vi "RT Main Test.vi"() -> ()   [LabVIEW 2020]
uses:
  <vilib>/Platform/TimedLoop/XDataNode/timing_clust.ctl
  <vilib>/Platform/TimedLoop/XDataNode/nitl_modes.ctl
  <vilib>/Platform/TimedLoop/XDataNode/wakeup.ctl
  Type Definitions/Payload Class.ctl
  Type Definitions/Enumerated Constants/Software Monitor.ctl
  Type Definitions/Queue Monitor.ctl
  Type Definitions/Telemetry TCP State.ctl
  Type Definitions/Enum - System State.ctl
  Type Definitions/Data Frame.ctl
  Type Definitions/Data Frame Header.ctl
  SubVIs/Compute CRC32.vi
  <vilib>/platform/TimedLoop/XDataNode/XDataNode.xnode
  <vilib>/Platform/TimedLoop/XDataNode/XDNodeRunTimeDep.lvlib
panel:
  out "error out":errorcluster
  out "Remote Address":string
  out "Remote Port":u16
  out "Frames Sent":i32
  out "Bytes Sent":i32
  out "Is Connected":bool
  out "Linux Standard Out":string
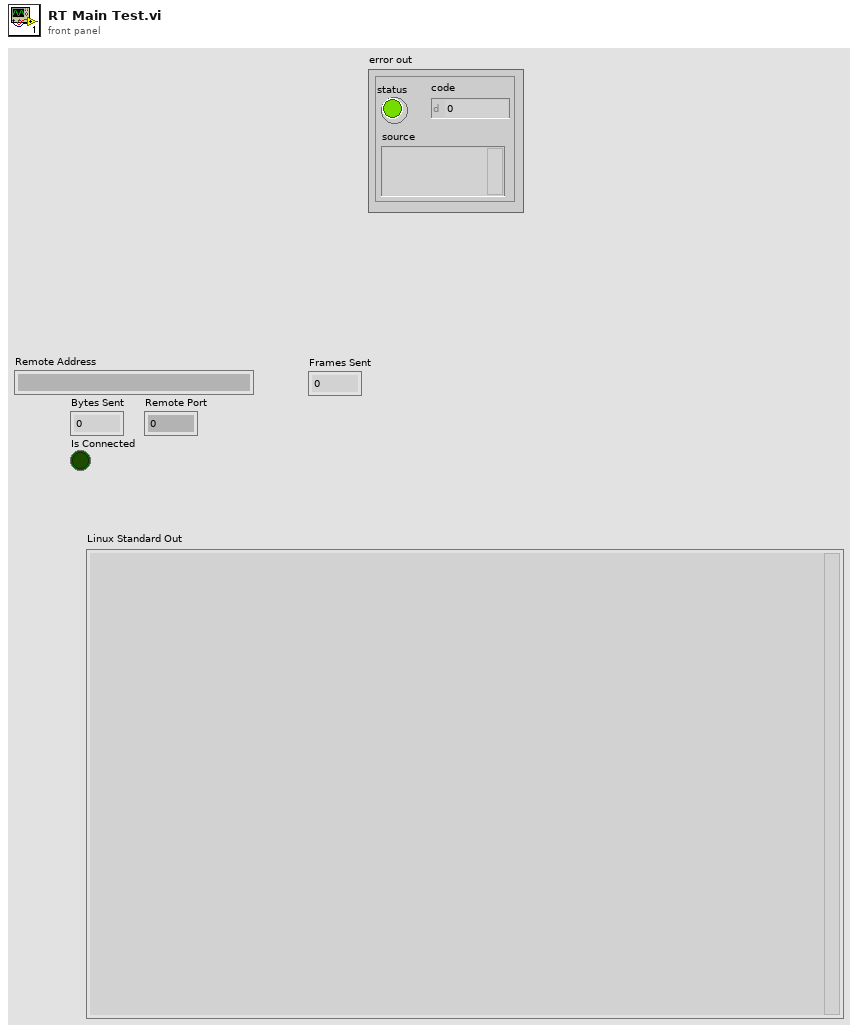
[diagram p1: front panel]
types:
  T1 = typedef "XDNodeRunTimeDep.lvlib/timing_clust.ctl" = cluster{"Expected End [f-1]":u64, "Actual End [f-1]":u64, "Finished Late? [f-1]":bool, "Expected End [i-1]":u64, "Actual End [i-1]":u64, "Finished Late? [i-1]":bool, "Expected Start [i]":u64, "Actual Start [i]":u64, "Expected Start [f]":u64, "Actual Start [f]":u64, "Source Name":string, "Structure Name":string, "Period":i64, "Deadline":i64, "Offset":i64, "Start":i64, "Priority":i32, "Timeout":i32, "Mode":T2, "Wakeup Reason":T3, "Error":errorcluster, "Source Type":string, "Secondary Source Type":string, "Global End Time":u64, "Global Start Time":u64, "Frame Duration":u64, "Iteration Duration":u64, "Assigned CPU":i32, "I/O Scan Engine Mode":u32}
  T2 = typedef "XDNodeRunTimeDep.lvlib/nitl_modes.ctl" = enum32{"No Change", "Process missed periods, maintain original phase", "Discard missed periods, maintain original phase", "Process missed periods, ignore original phase", "Discard missed periods, ignore original phase"}
  T3 = typedef "XDNodeRunTimeDep.lvlib/wakeup.ctl" = enum32{"Normal", "Aborted", "Asynchronous wakeup", "Timing source error", "Timed loop error", "Timeout"}
  T4 = typedef "Software Monitor.ctl" = enum16{"Internet Connection Monitor", "CPU Monitor", "Archive Monitor", "Memory Monitor", "Queue Monitor", "RTOS Update", "RTOS Monitor"}
  T5 = typedef "Payload Class.ctl" = enum16{"System State", "Parameters", "Metadata", "Software Monitor", "Data", "Commands"}
  T6 = typedef "Queue Monitor.ctl" = cluster{"Queue Name":string, "Max Queue Size":i32, "Pending Remove":i32, "Pending Insert":i32, "Elements in Queue":i32}
  T7 = typedef "Data Frame.ctl" = cluster{"Frame Header":T8, "Payload":string, "CRC":u32}
  T8 = typedef "Data Frame Header.ctl" = cluster{"Sync":u32, "Time":dbl, "Nanosecond Counter":i64, "Payload Class":T5, "Payload ID":u16, "Counter":u32, "Options":u32, "Source":i32, "Destination":i32}
  T9 = typedef "Enum - System State.ctl" = enum16{"System Time", "Telemetry TCP State", "Writeable Drive State", "Command TCP State", "Network Adapter State", "Discovery Engine State", "Disk State"}
  T10 = typedef "Telemetry TCP State.ctl" = cluster{"Is Connected":bool, "Remote Address":string, "Remote Port":u16, "Total Frames Sent":i32, "Total Bytes Sent":i32}
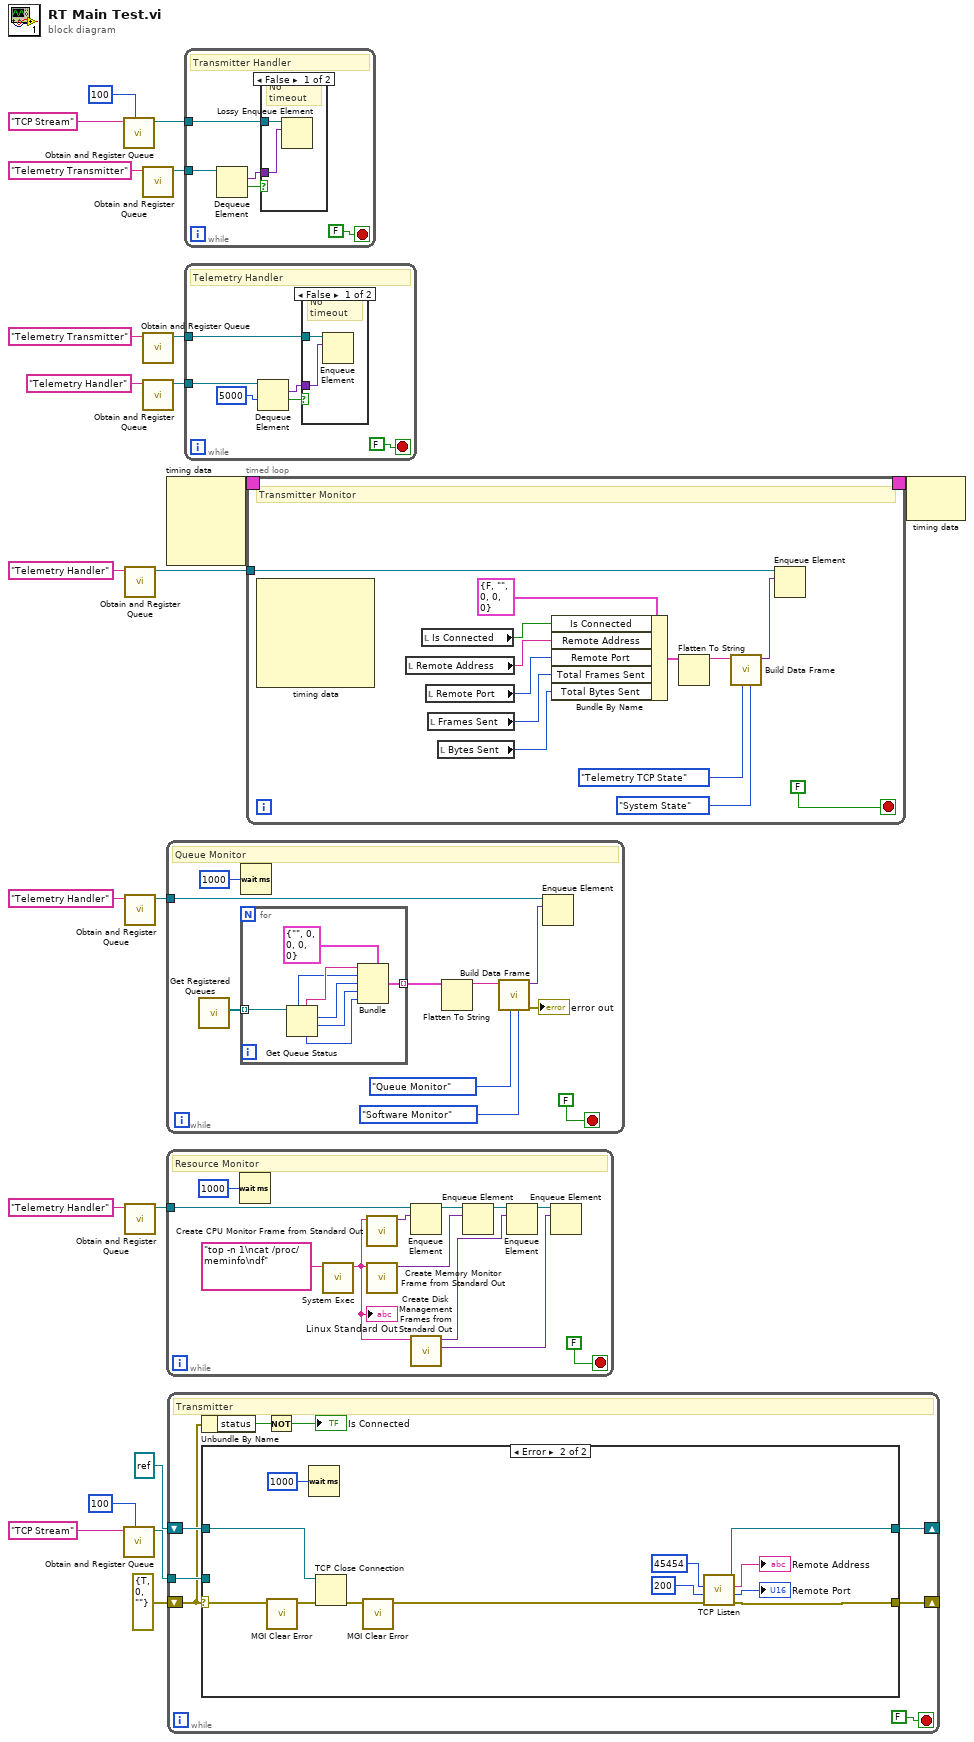
[diagram p0: block diagram]
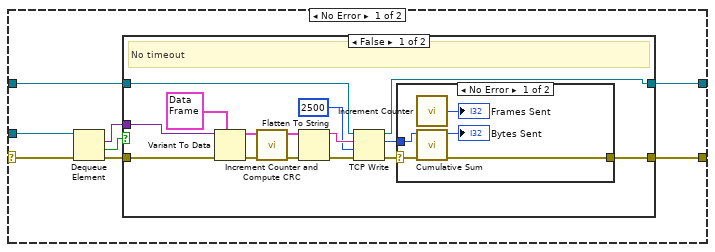
[diagram p3: hidden frame]
diagram:
  n1 = call "Obtain and Register Queue.vi"("max queue size (-1, unlimited)"=100, "name (unnamed)"="TCP Stream") -> ("Queue Out"=w2:refnum<queue>)  [unwired: 6 in, 3 out]
  n2 = call "Obtain and Register Queue.vi"("max queue size (-1, unlimited)"=100, "name (unnamed)"="TCP Stream") -> ("Queue Out"=w9:refnum<queue>)  [unwired: 6 in, 3 out]
  n3 = call "Obtain and Register Queue.vi"("name (unnamed)"="Telemetry Handler") -> ("Queue Out"=w7:refnum<queue>)  [unwired: 7 in, 3 out]
  n4 = call "Obtain and Register Queue.vi"("name (unnamed)"="Telemetry Handler") -> ("Queue Out"=w14:refnum<queue>)  [unwired: 7 in, 3 out]
  n5 = call "Obtain and Register Queue.vi"("name (unnamed)"="Telemetry Handler") -> ("Queue Out"=w16:refnum<queue>)  [unwired: 7 in, 3 out]
  n6 = call "Obtain and Register Queue.vi"("name (unnamed)"="Telemetry Transmitter") -> ("Queue Out"=w4:refnum<queue>)  [unwired: 7 in, 3 out]
  n7 = call "Obtain and Register Queue.vi"("name (unnamed)"="Telemetry Transmitter") -> ("Queue Out"=w20:refnum<queue>)  [unwired: 7 in, 3 out]
  n8 = call "Obtain and Register Queue.vi"("name (unnamed)"="Telemetry Handler") -> ("Queue Out"=w19:refnum<queue>)  [unwired: 7 in, 3 out]
  n9 = node-c288() -> (w22:T1)  [unwired: 4 in]
  n10 = while {
    tunnel: w14 -> [w26]
    stop <- FALSE stop-if-true
    # "Queue Monitor"
    n11 = call "Get Registered Queues.vi"() -> ("Queue References"=w31:refnum<queue>[])  [unwired: 9 in, 2 out]
    n12 = Wait (ms)(milliseconds to wait=u32 1000) -> ()  [unwired: 1 out]
    n13 = for {
      tunnel: w31 -> [w40] mode=indexing
      tunnel: [w34] -> w27 mode=indexing
      n14 = Get Queue Status(queue=w40) -> (queue name=w39:string, max queue size=w38:i32, # pending remove=w37:i32, # pending insert=w36:i32, # elements in queue=w35:i32)  [unwired: 2 in, 3 out]
      n15 = Bundle(cluster=T6 {"Queue Name"="", "Max Queue Size"=0, "Pending Remove"=0, "Pending Insert"=0, "Elements in Queue"=0}, "Queue Name"=w39, "Max Queue Size"=w38, "Pending Remove"=w37, "Pending Insert"=w36, "Elements in Queue"=w35) -> (w34:T6)
    }
    n16 = Flatten To String(anything=w27) -> (data string=w30:string)  [unwired: 3 in, 2 out]
    n17 = call "Build Data Frame.vi"("Payload Class (Data)"=Payload_Class."Software Monitor", "Payload ID (0)"=Software_Monitor."Queue Monitor", "Payload (Empty String)"=w30) -> ("error out"=→"error out":errorcluster, "Frame"=w25:variant)  [unwired: 7 in]
    n18 = Enqueue Element(queue=w26, element=w25) -> ()  [unwired: 2 in, 3 out]
  }
  n19 = while {
    tunnel: w16 -> [w50]
    stop <- FALSE stop-if-true
    # "Resource Monitor"
    n20 = Wait (ms)(milliseconds to wait=u32 1000) -> ()  [unwired: 1 out]
    n21 = call <vilib>:"System Exec.vi"("command line"="top -n 1\ncat /proc/meminfo\ndf") -> ("standard output"=w42:string)  [unwired: 7 in, 3 out]
    "Linux Standard Out" <- w42
    n22 = call "Create CPU Monitor Frame from Standard Out.vi"("Standard Output"=w42) -> ("Frame"=w51:variant)  [unwired: 10 in]
    n23 = call "Create Memory Monitor Frame from Standard Out.vi"("Starndard Output"=w42) -> ("Frame"=w46:variant)  [unwired: 10 in]
    n24 = Enqueue Element(queue=w50, element=w51) -> (queue out=w49:refnum<queue>)  [unwired: 2 in, 2 out]
    n25 = call "Create Disk Management Frames from Standard Out.vi"("Standard Output"=w42) -> ("Writeable Drives Frame"=w44:variant, "Disk Management Frame"=w47:variant)  [unwired: 9 in]
    n26 = Enqueue Element(queue=w49, element=w46) -> (queue out=w48:refnum<queue>)  [unwired: 2 in, 2 out]
    n27 = Enqueue Element(queue=w48, element=w47) -> (queue out=w45:refnum<queue>)  [unwired: 2 in, 2 out]
    n28 = Enqueue Element(queue=w45, element=w44) -> ()  [unwired: 2 in, 3 out]
  }
  n29 = while {
    shift-right: [w60] -> _
    shift-left: errorcluster {"status"=TRUE, "code"=0, "source"=""} ("error out") -> [w55]
    shift-right: [w56] -> _
    shift-left: refnum<k5> refnum ("connection ID") -> [w59]
    tunnel: w9 -> [w58]
    stop <- FALSE stop-if-true
    # "Transmitter"
    n30 = Unbundle By Name(w55) -> ("status"=w54:bool)
    n31 = case shown="Error" w55 {
      selector: w55 -> [w67 w93]
      tunnel: [w62 w98] -> w60
      tunnel: [w63 w100] -> w56
      tunnel: w59 -> [w66 w102]
      tunnel: w58 -> [w68 _]
      frame No Error {
        n32 = Dequeue Element(queue=w68, error in (no error)=w67) -> (element=w65:variant, timed out?=w61:bool, error out=w64:errorcluster)  [unwired: 1 in, 1 out]
        n33 = case shown="False" w61 {
          tunnel: w66 -> [w83 w90]
          tunnel: w65 -> [w81 _]
          tunnel: w64 -> [w78 w91]
          tunnel: [w74 w90] -> w63
          tunnel: [w70 w91] -> w62
          frame False {
            # "No timeout"
            n34 = Variant To Data(error in=w78, type=T7 {"Frame Header"={"Sync"=0, "Time"=0.0, "Nanosecond Counter"=0, "Payload Class"=enum."System State", "Payload ID"=0, "Counter"=0, "Options"=0, "Source"=0, "Destination"=0}, "Payload"="", "CRC"=0} ("Frame"), Variant=w81) -> (data=w82:T7, error out=w77:errorcluster)
            n35 = call "Increment Counter and Compute CRC.vi"("error in (no error)"=w77, "Frame In"=w82) -> ("error out"=w76:errorcluster, "Frame Out"=w72:T7)  [unwired: 8 in]
            n36 = Flatten To String(anything=w72, error in (no error)=w76) -> (data string=w79:string, error out=w75:errorcluster)  [unwired: 2 in, 1 out]
            n37 = TCP Write(connection ID=w83, data in=w79, error in (no error)=w75, 9:2500 ("timeout ms (25000)")) -> (connection ID out=w74:refnum<k5>, bytes written=w73:i32, error out=w69:errorcluster)
            n38 = case shown="No Error" w69 {
              selector: w69 -> [w85 w89]
              tunnel: w73 -> [w86 _]
              tunnel: [w84 w89] -> w70
              frame No Error {
                n39 = call "Increment Counter.vi"() -> ("Count"=→"Frames Sent":i32)  [unwired: 5 in]
                n40 = call "Cumulative Sum.vi"("error in (no error)"=w85, "Value In"=w86) -> ("error out"=w84:errorcluster, "Cumulative Sum"=→"Bytes Sent":i32)  [unwired: 8 in]
              }
              frame Error {
              }
            }
          }
          frame True {
            # "Timed out"
          }
        }
      }
      frame Error {
        n41 = call <userlib>:"MGI Clear Error.vi"("Error In"=w93) -> ("Error Out"=w92:errorcluster)  [unwired: 6 in]
        n42 = Wait (ms)(milliseconds to wait=u32 1000) -> ()  [unwired: 1 out]
        n43 = TCP Close Connection(connection ID=w102, error in (no error)=w92) -> (error out=w101:errorcluster)  [unwired: 1 in, 1 out]
        n44 = call <userlib>:"MGI Clear Error.vi"("Error In"=w101) -> ("Error Out"=w99:errorcluster)  [unwired: 6 in]
        n45 = call <vilib>:"TCP Listen.vi"("error in (no error)"=w99, "timeout ms (wait forever: -1)"=200, "port"=u16 45454) -> ("error out"=w98:errorcluster, "remote port"=→"Remote Port":u16, "remote address"=→"Remote Address":string, "connection ID"=w100:refnum<k5>)  [unwired: 4 in, 1 out]
      }
    }
    n46 = Not(x=w54) -> (.not. x?=→"Is Connected":bool)
  }
  n47 = while {
    tunnel: w4 -> [w108]
    tunnel: w2 -> [w106]
    stop <- FALSE stop-if-true
    # "Transmitter Handler"
    n48 = Dequeue Element(queue=w108) -> (element=w105:variant, timed out?=w104:bool)  [unwired: 2 in, 2 out]
    n49 = case shown="False" w104 {
      tunnel: w106 -> [w110 _]
      tunnel: w105 -> [w109 _]
      frame False {
        # "No timeout"
        n50 = Lossy Enqueue Element(queue=w110, element=w109) -> ()  [unwired: 1 in, 4 out]
      }
      frame True {
        # "Timed out"
      }
    }
  }
  n51 = while {
    tunnel: w19 -> [w116]
    tunnel: w20 -> [w114]
    stop <- FALSE stop-if-true
    # "Telemetry Handler"
    n52 = Dequeue Element(queue=w116, timeout in ms (-1)=5000) -> (element=w113:variant, timed out?=w112:bool)  [unwired: 1 in, 2 out]
    n53 = case shown="False" w112 {
      tunnel: w114 -> [w118 _]
      tunnel: w113 -> [w117 _]
      frame False {
        # "No timeout"
        n54 = Enqueue Element(queue=w118, element=w117) -> ()  [unwired: 2 in, 3 out]
      }
      frame True {
        # "Timed out"
      }
    }
  }
  n55 = timed-loop {
    timing: w22 -> [_]
    timing-out: [_] -> w21
    tunnel: w7 -> [w126]
    stop <- FALSE stop-if-true
    # "Transmitter Monitor"
    n56 = node-c288() -> ()  [unwired: 1 in, 6 out]
    n57 = local read "Remote Address"() -> (w123:string)
    n58 = local read "Is Connected"() -> (w119:bool)
    n59 = local read "Remote Port"() -> (w122:u16)
    n60 = local read "Frames Sent"() -> (w121:i32)
    n61 = local read "Bytes Sent"() -> (w120:i32)
    n62 = Bundle By Name(cluster=T10 {"Is Connected"=FALSE, "Remote Address"="", "Remote Port"=0, "Total Frames Sent"=0, "Total Bytes Sent"=0} ("Cluster"), "Is Connected"=w119, "Remote Address"=w123, "Remote Port"=w122, "Total Frames Sent"=w121, "Total Bytes Sent"=w120) -> (w125:T10)
    n63 = Flatten To String(anything=w125) -> (data string=w128:string)  [unwired: 3 in, 2 out]
    n64 = call "Build Data Frame.vi"("Payload Class (Data)"=Payload_Class."System State", "Payload ID (0)"=Enum_-_System_State."Telemetry TCP State" ("System State"), "Payload (Empty String)"=w128) -> ("Frame"=w127:variant)  [unwired: 7 in, 1 out]
    n65 = Enqueue Element(queue=w126, element=w127) -> ()  [unwired: 2 in, 3 out]
  }
  n66 = node-c288(w21) -> ()  [unwired: 1 out]
